vi "Add Calibration.vi"() -> ()   [LabVIEW 2020]
panel:
  in  "Temperature":dbl
  in  "Calibration Date":timestamp format="%<%x>T"
  in  "Serial Number":string
  in  "Model":string
  in  "Vendor":string
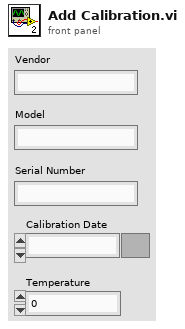
[diagram p1: front panel]
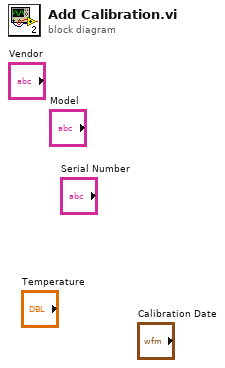
[diagram p0: block diagram]
diagram:
